vi "Unconstrained Power Fit.vi"(0 "Y":dbl[](array[numeric]), 5 "X":dbl[](array[numeric]), 7 "Weight":dbl[](array[numeric]), 9 "tolerance":dbl=0.0001 format="%#_3g", 11 "method":T1 items=["Least Square", "Least Absolute Residual", "Bisquare"]) -> (4 "Best Power Fit":dbl[](array[numeric]), 6 "amplitude":dbl, 8 "power":dbl, 14 "residue":dbl, 15 "error":i32)   [LabVIEW 2020, in "NI_AALPro.lvlib"]
doc: "Returns the power fit of a data set (<B>X</B>, <B>Y</B>) using the Least Square, Least Absolute Residual, or Bisquare method."
uses:
  NI_AALPro.lvlib
  Curve Fitting Criteria.ctl
panel:
  # "Power Fit"
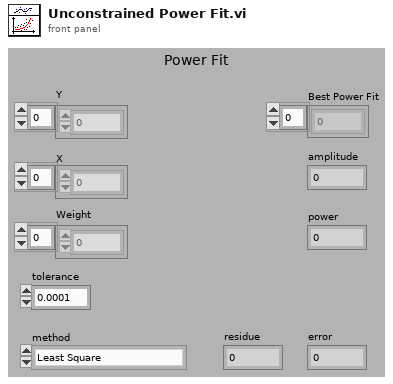
[diagram p1: front panel]
types:
  T1 = typedef "NI_AALPro.lvlib/Curve Fitting Criteria.ctl" = u16
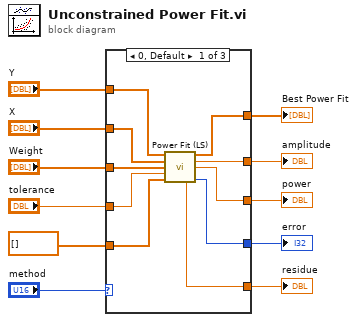
[diagram p0: block diagram]
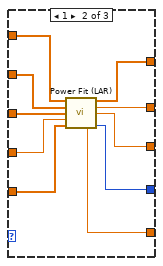
[diagram p2: hidden frame]
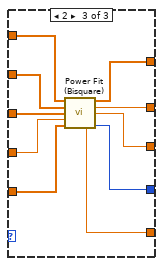
[diagram p3: hidden frame]
diagram:
  n1 = case shown="0, Default" "method" {
    tunnel: "Y" -> [w21 w31 w41]
    tunnel: "X" -> [w20 w30 w40]
    tunnel: "Weight" -> [w19 w29 w39]
    tunnel: "tolerance" -> [w18 w28 w38]
    tunnel: dbl[] [] ("array") -> [w17 w27 w37]
    tunnel: [w16 w22 w36] -> w6
    tunnel: [w15 w26 w35] -> w5
    tunnel: [w14 w25 w34] -> w4
    tunnel: [w13 w24 w33] -> w3
    tunnel: [w12 w23 w32] -> w2
    frame 0, Default {
      n2 = call "Power Fit (LS).vi"("Y"=w21, "X"=w20, "Weight"=w19, "tolerance"=w18, "Initial Coefficients"=w17) -> ("Best Power Fit"=w15:dbl[], "amplitude"=w14:dbl, "power"=w13:dbl, "residue"=w16:dbl, "error"=w12:i32)  [unwired: 6 out]
    }
    frame 1 {
      n3 = call "Power Fit (LAR).vi"("Y"=w31, "X"=w30, "Weight"=w29, "tolerance"=w28, "Initial Coefficients"=w27) -> ("Best Power Fit"=w26:dbl[], "amplitude"=w25:dbl, "power"=w24:dbl, "residue"=w22:dbl, "error"=w23:i32)  [unwired: 6 out]
    }
    frame 2 {
      n4 = call "Power Fit (Bisquare).vi"("Y"=w41, "X"=w40, "Weight"=w39, "tolerance"=w38, "Initial Coefficients"=w37) -> ("Best Power Fit"=w35:dbl[], "amplitude"=w34:dbl, "power"=w33:dbl, "residue"=w36:dbl, "error"=w32:i32)  [unwired: 6 out]
    }
  }
  "amplitude" <- w4
  "power" <- w3
  "error" <- w2
  "Best Power Fit" <- w5
  "residue" <- w6
